vi "Fano Factor Zero Finder f(x) 1D.vi"(4 "data":variant, 5 "x":dbl) -> (2 "f(x)":dbl)   [LabVIEW 2021, in "Math.lvlib"]
uses:
  Math Fano Factor Zero Finder Data.ctl
  37d6fc3c-26f2-4b22-9b93-2ffa8a75d867.vi
  Math.lvlib
  <vilib>/gmath/NI_Gmath.lvlib
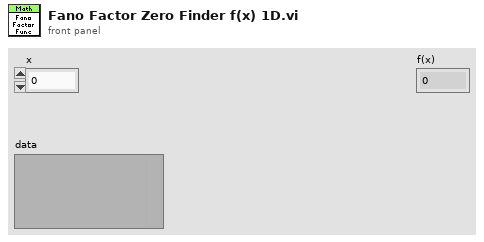
[diagram p1: front panel]
types:
  T1 = typedef "Math.lvlib/Math Fano Factor Zero Finder Data.ctl" = cluster{"Data":dbl[], "Fit":dbl[]}
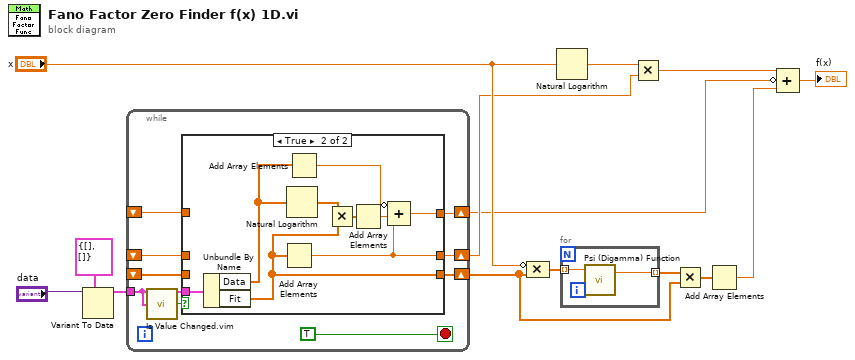
[diagram p0: block diagram]
diagram:
  n1 = Variant To Data(type=T1 {"Data"=[], "Fit"=[]} ("Fano Factor Optimization Parameters"), Variant="data") -> (data=w12:T1)  [unwired: 1 in, 1 out]
  n2 = while {
    tunnel: w12 -> [w20]
    shift-right: [w19] -> w6
    shift-left: _ -> [w21]
    shift-right: [w18] -> w9
    shift-left: _ -> [w15]
    shift-right: [w17] -> w2
    shift-left: _ -> [w16]
    stop <- TRUE stop-if-true
    n3 = call "Is Value Changed.vim"("value"=w20) -> ("changed or first call?"=w22:bool)
    n4 = case shown="True" w22 {
      tunnel: w21 -> [w24 _]
      tunnel: w20 -> [_ w35]
      tunnel: [w24 w33] -> w19
      tunnel: [w25 w30] -> w18
      tunnel: [w26 w27] -> w17
      tunnel: w16 -> [w26 _]
      tunnel: w15 -> [w25 _]
      frame False {
      }
      frame True {
        n5 = Unbundle By Name(w35) -> ("Data"=w31:dbl[], "Fit"=w33:dbl[])
        n6 = Add Array Elements(numeric array=w33) -> (sum=w30:dbl)
        n7 = Natural Logarithm(1:w31) -> (0:w34:dbl[])
        n8 = Add Array Elements(numeric array=w31) -> (sum=w29:dbl)
        n9 = Multiply(x=w34, y=w33) -> (x*y=w32:dbl[])
        n10 = Add Array Elements(numeric array=w32) -> (sum=w28:dbl)
        n11 = Compound Arithmetic op=ADD(invert w29, w28, w30) -> (w27:dbl)
      }
    }
  }
  n12 = Compound Arithmetic op=MULTIPLY(invert "x", w6) -> (w8:dbl[])
  n13 = Natural Logarithm(1:"x") -> (0:w11:dbl)
  n14 = for {
    tunnel: w8 -> [w37] mode=indexing
    tunnel: [w36] -> w7 mode=indexing
    n15 = call <vilib>:"Psi (Digamma) Function.vi"("x"=w37) -> ("y(x)"=w36:dbl)  [unwired: 2 in]
  }
  n16 = Multiply(x=w11, y=w9) -> (x*y=w5:dbl)
  n17 = Multiply(x=w7, y=w6) -> (x*y=w4:dbl[])
  n18 = Add Array Elements(numeric array=w4) -> (sum=w3:dbl)
  n19 = Compound Arithmetic op=ADD(w5, invert w2, w3) -> (→"f(x)":dbl)
